vi "SubVI_UserSliderCursor.vi"(6 "Axes colour":u32(colorbox)=16711680, 8 "error in (no error)":errorcluster, 9 "Image RefNum In":T1, 10 "Y slider refnum":refnum<vi>, 11 "X slider refnum":refnum<vi>) -> (0 "error out":errorcluster, 2 "Image Refnum out":T1, 3 "Cross Point":cluster{"X coordinate":dbl, "Y coordinate":dbl})   [LabVIEW 2016]
uses:
  <vilib>/vision/Image Controls.llb/IMAQ Image.ctl
panel:
  # "This subVI takes input from a pair of \nsliders to display axes on an image. \nThe Cross Point provides the \n(x,y) coordinates of the intersection\nof the two axes (in pixel units)"
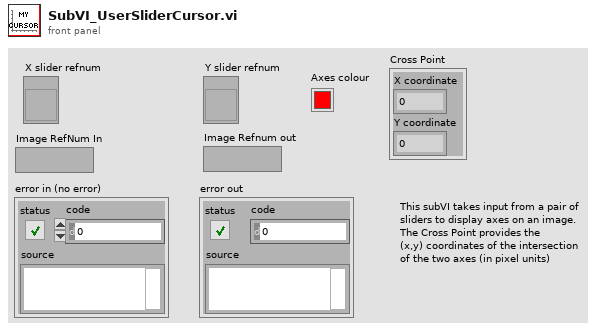
[diagram p1: front panel]
types:
  T1 = typedef "IMAQ Image.ctl" = refnum<image>
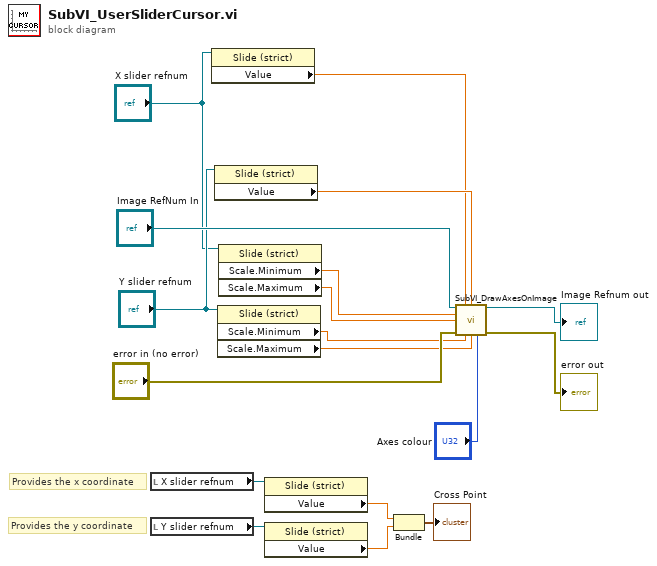
[diagram p0: block diagram]
diagram:
  # "Provides the x coordinate"
  # "Provides the y coordinate"
  n1 = local read "X slider refnum"() -> (w5:refnum<vi>)
  n2 = local read "Y slider refnum"() -> (w4:refnum<vi>)
  n3 = property class="Slide (strict)"(reference="X slider refnum") -> ("Value"=w6:dbl)  [unwired: 1 in, 2 out]
  n4 = property class="Slide (strict)"(reference="Y slider refnum") -> ("Value"=w7:dbl)  [unwired: 1 in, 2 out]
  n5 = property on="Property Node" class="Slide (strict)"(reference="Y slider refnum") -> ("Scale.Minimum"=w10:dbl, "Scale.Maximum"=w11:dbl)  [unwired: 1 in, 2 out]
  n6 = property on="Property Node" class="Slide (strict)"(reference="X slider refnum") -> ("Scale.Minimum"=w8:dbl, "Scale.Maximum"=w9:dbl)  [unwired: 1 in, 2 out]
  n7 = property class="Slide (strict)"(reference=w5) -> ("Value"=w2:dbl)  [unwired: 1 in, 2 out]
  n8 = property class="Slide (strict)"(reference=w4) -> ("Value"=w1:dbl)  [unwired: 1 in, 2 out]
  n9 = Bundle("Value"=w2, "Value"=w1) -> (→"Cross Point":cluster{"Value":dbl, "Value":dbl})  [unwired: 1 in]
  n10 = call "SubVI_DrawAxesOnImage.vi"("Image Refnum in"="Image RefNum In", "X Value"=w6, "Y Value"=w7, "X Minimum"=w8, "X Maximum"=w9, "error in (no error)"="error in (no error)", "Y Minimum"=w10, "Y Maximum"=w11, "Axes colour"="Axes colour") -> ("Image Refnum out"=→"Image Refnum out":T1, "error out"=→"error out":errorcluster)  [unwired: 5 in]
